vi "gantry移動定位_六邊形(外切圓)(旋轉).vi"() -> ()   [LabVIEW 2016]
uses:
  Classes/Controller/Motion/A3200 Folder/A3200.lvclass
panel:
  in  "旋轉角度":dbl
  out "點座標":dbl[][](array[numeric])
  in  "外切圓半徑":dbl=100.0
  in  "中心點座標":dbl[](array[numeric])
  out "Final Position":dbl[](array[numeric])
  out "Initial position":dbl[](array[numeric])
  in  "Speed (mm/s)":dbl=40.0
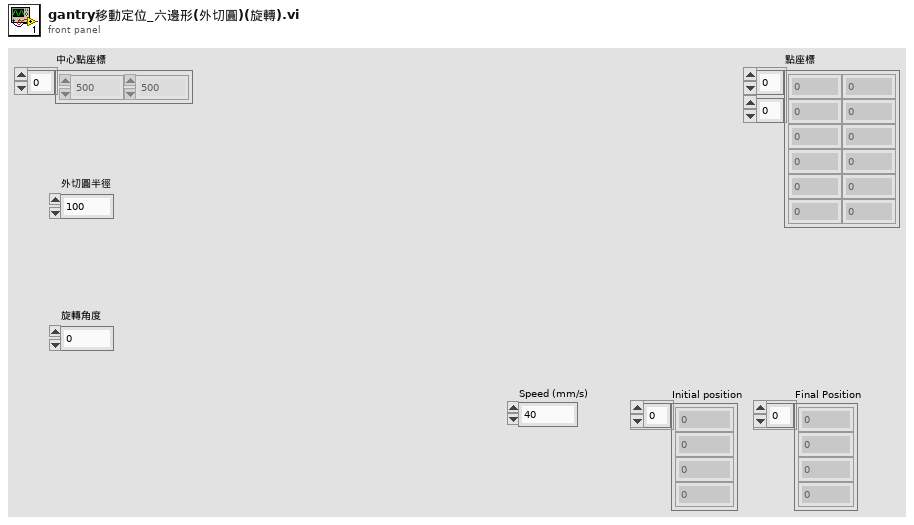
[diagram p1: front panel]
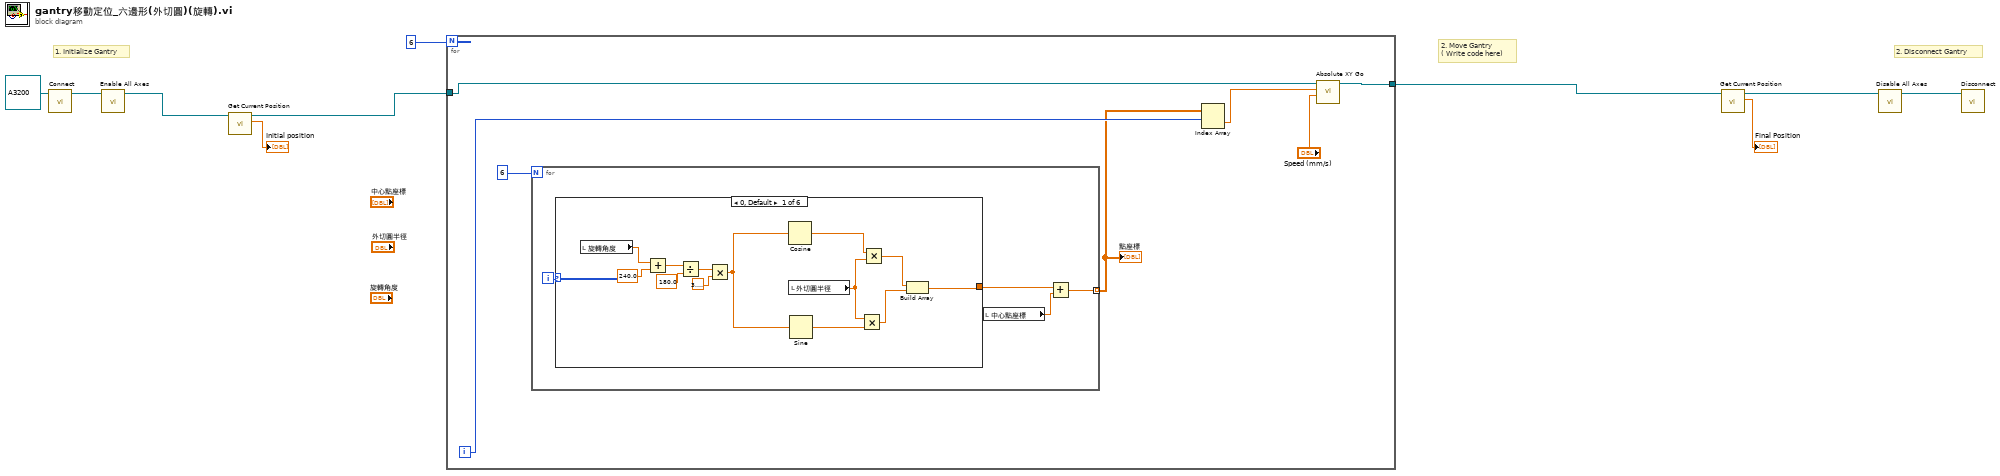
[diagram p0: block diagram]
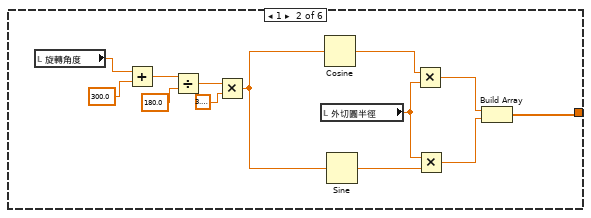
[diagram p2: hidden frame]
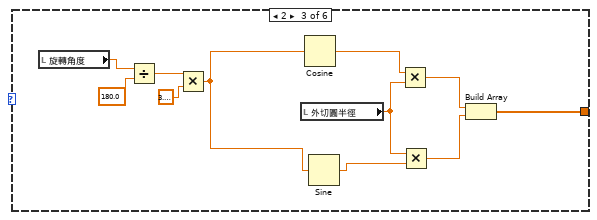
[diagram p3: hidden frame]
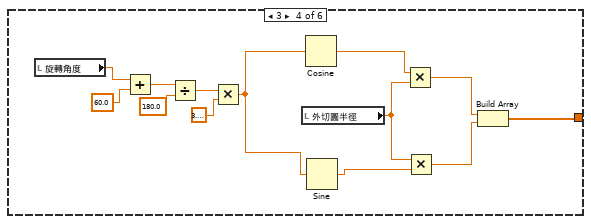
[diagram p4: hidden frame]
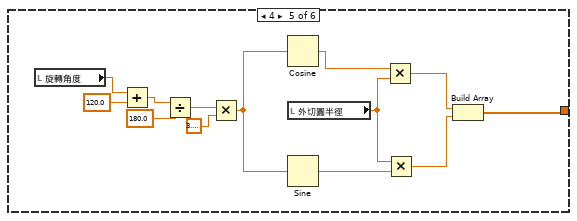
[diagram p5: hidden frame]
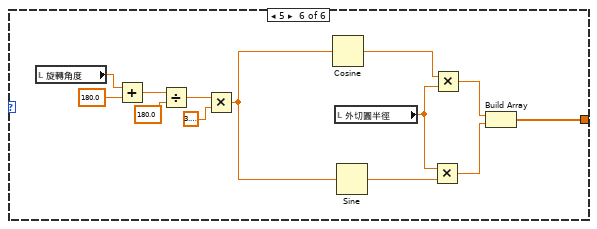
[diagram p6: hidden frame]
diagram:
  # "1. Initialize Gantry"
  # "2. Disconnect Gantry"
  # "2. Move Gantry \n( Write code here)"
  n1 = call-dynamic "Connect.vi"("Gantry in"=refnum<class "A3200.lvclass"> refnum ("A3200.lvclass")) -> ("Gantry out"=w5:refnum<class "A3200.lvclass">)  [unwired: 9 in, 1 out]
  n2 = call-dynamic "Enable All Axes.vi"("A3200 in"=w5) -> ("A3200 out"=w4:refnum<class "A3200.lvclass">)  [unwired: 9 in, 1 out]
  n3 = call-dynamic "Get Current Position.vi"("Gantry in"=w4) -> ("XYZTheta Out"=→"Initial position":dbl[], "Gantry out"=w3:refnum<class "A3200.lvclass">)  [unwired: 8 in, 1 out]
  n4 = for {
    N: 6 -> [_]
    tunnel: w3 -> [w15]
    tunnel: [w14] -> w2
    i -> [w17]
    n5 = for {
      N: 6 -> [_]
      tunnel: [w19] -> w12 mode=indexing
      i -> [w21]
      n6 = case shown="0, Default" w21 {
        tunnel: [w34 w35 w48 w59 w72 w97] -> w18
        frame 0, Default {
          n7 = local read "旋轉角度"() -> (w33:dbl)
          n8 = Add(x=w33, y=240.0) -> (x+y=w31:dbl)
          n9 = Divide(x=w31, y=180.0) -> (x/y=w29:dbl)
          n10 = Multiply(x=w29, y=3.141592653589793) -> (x*y=w25:dbl)
          n11 = Cosine(x=w25) -> (cos(x)=w27:dbl)
          n12 = local read "外切圓半徑"() -> (w23:dbl)
          n13 = Sine(x=w25) -> (sin(x)=w24:dbl)
          n14 = Multiply(x=w23, y=w24) -> (x*y=w22:dbl)
          n15 = Multiply(x=w27, y=w23) -> (x*y=w26:dbl)
          n16 = Build Array(w26, w22) -> (w34:dbl[])
        }
        frame 1 {
          n17 = local read "旋轉角度"() -> (w47:dbl)
          n18 = Add(x=w47, y=300.0) -> (x+y=w45:dbl)
          n19 = Divide(x=w45, y=180.0) -> (x/y=w43:dbl)
          n20 = Multiply(x=w43, y=3.141592653589793) -> (x*y=w40:dbl)
          n21 = local read "外切圓半徑"() -> (w38:dbl)
          n22 = Cosine(x=w40) -> (cos(x)=w41:dbl)
          n23 = Sine(x=w40) -> (sin(x)=w39:dbl)
          n24 = Multiply(x=w41, y=w38) -> (x*y=w36:dbl)
          n25 = Multiply(x=w38, y=w39) -> (x*y=w37:dbl)
          n26 = Build Array(w36, w37) -> (w35:dbl[])
        }
        frame 2 {
          n27 = local read "旋轉角度"() -> (w58:dbl)
          n28 = Divide(x=w58, y=180.0) -> (x/y=w56:dbl)
          n29 = Multiply(x=w56, y=3.141592653589793) -> (x*y=w53:dbl)
          n30 = local read "外切圓半徑"() -> (w51:dbl)
          n31 = Cosine(x=w53) -> (cos(x)=w54:dbl)
          n32 = Sine(x=w53) -> (sin(x)=w52:dbl)
          n33 = Multiply(x=w54, y=w51) -> (x*y=w49:dbl)
          n34 = Multiply(x=w51, y=w52) -> (x*y=w50:dbl)
          n35 = Build Array(w49, w50) -> (w48:dbl[])
        }
        frame 3 {
          n36 = local read "旋轉角度"() -> (w71:dbl)
          n37 = Add(x=w71, y=60.0) -> (x+y=w69:dbl)
          n38 = Divide(x=w69, y=180.0) -> (x/y=w67:dbl)
          n39 = Multiply(x=w67, y=3.141592653589793) -> (x*y=w64:dbl)
          n40 = local read "外切圓半徑"() -> (w62:dbl)
          n41 = Cosine(x=w64) -> (cos(x)=w65:dbl)
          n42 = Sine(x=w64) -> (sin(x)=w63:dbl)
          n43 = Multiply(x=w65, y=w62) -> (x*y=w60:dbl)
          n44 = Multiply(x=w62, y=w63) -> (x*y=w61:dbl)
          n45 = Build Array(w60, w61) -> (w59:dbl[])
        }
        frame 4 {
          n46 = local read "旋轉角度"() -> (w84:dbl)
          n47 = Add(x=w84, y=120.0) -> (x+y=w82:dbl)
          n48 = Divide(x=w82, y=180.0) -> (x/y=w80:dbl)
          n49 = Multiply(x=w80, y=3.141592653589793) -> (x*y=w76:dbl)
          n50 = Cosine(x=w76) -> (cos(x)=w78:dbl)
          n51 = local read "外切圓半徑"() -> (w74:dbl)
          n52 = Sine(x=w76) -> (sin(x)=w75:dbl)
          n53 = Multiply(x=w78, y=w74) -> (x*y=w77:dbl)
          n54 = Multiply(x=w74, y=w75) -> (x*y=w73:dbl)
          n55 = Build Array(w77, w73) -> (w72:dbl[])
        }
        frame 5 {
          n56 = local read "旋轉角度"() -> (w96:dbl)
          n57 = Add(x=w96, y=180.0) -> (x+y=w94:dbl)
          n58 = Divide(x=w94, y=180.0) -> (x/y=w92:dbl)
          n59 = Multiply(x=w92, y=3.141592653589793) -> (x*y=w88:dbl)
          n60 = Cosine(x=w88) -> (cos(x)=w90:dbl)
          n61 = local read "外切圓半徑"() -> (w86:dbl)
          n62 = Sine(x=w88) -> (sin(x)=w87:dbl)
          n63 = Multiply(x=w86, y=w87) -> (x*y=w85:dbl)
          n64 = Multiply(x=w90, y=w86) -> (x*y=w89:dbl)
          n65 = Build Array(w89, w85) -> (w97:dbl[])
        }
      }
      n66 = local read "中心點座標"() -> (w20:dbl[])
      n67 = Add(x=w18, y=w20) -> (x+y=w19:dbl[])
    }
    "點座標" <- w12
    n68 = Index Array(array=w12, index (row)=w17) -> (element=w11:dbl[])  [unwired: 1 in]
    n69 = call-dynamic "Absolute XY Go.vi"("Speed"="Speed (mm/s)", "XY"=w11, "Gantry in"=w15) -> ("Gantry out"=w14:refnum<class "A3200.lvclass">)  [unwired: 7 in, 1 out]
  }
  n70 = call-dynamic "Get Current Position.vi"("Gantry in"=w2) -> ("XYZTheta Out"=→"Final Position":dbl[], "Gantry out"=w8:refnum<class "A3200.lvclass">)  [unwired: 8 in, 1 out]
  n71 = call-dynamic "Disable All Axes.vi"("Gantry in"=w8) -> ("Gantry out"=w9:refnum<class "A3200.lvclass">)  [unwired: 9 in, 1 out]
  n72 = call-dynamic "Disconnect.vi"("Gantry in"=w9) -> ()  [unwired: 9 in, 1 out]
